vi "Set WordWrap.vi"(8 "error in":errorcluster, 10 "WordWrap":bool, 11 "View in":refnum<class "Cell View.lvclass">) -> (0 "error out":errorcluster, 3 "View out":refnum<class "Cell View.lvclass">)   [LabVIEW 2024, in "SourceGrid.lvlib" / "Cell View.lvclass"]
uses:
  Cell View.lvclass
  Cell View.lvclass/Cell View.ctl
  D:/git/Sourcegrid-LabVIEW/dll/SourceGrid.dll
  dll/SourceGrid.dll
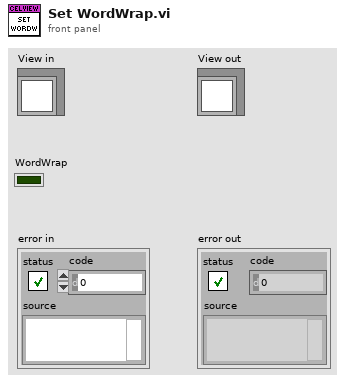
[diagram p1: front panel]
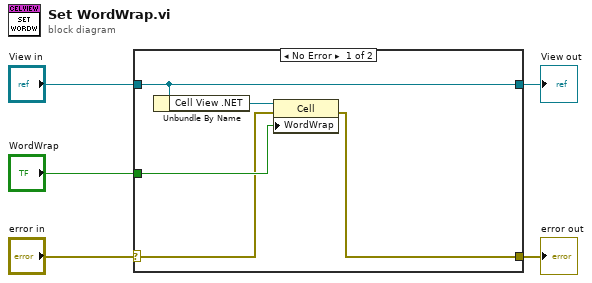
[diagram p0: block diagram]
diagram:
  n1 = case shown="No Error" "error in" {
    selector: "error in" -> [w7 w11]
    tunnel: [w6 w11] -> w4
    tunnel: [w10 w12] -> w2
    tunnel: "View in" -> [w10 w12]
    tunnel: "WordWrap" -> [w8 _]
    frame No Error {
      n2 = Unbundle By Name(w10) -> ("Cell View .NET"=w9:refnum<k24>)
      n3 = property class="Cell"(reference=w9, error in=w7, "WordWrap"=w8) -> (error out=w6:errorcluster)  [unwired: 1 out]
    }
    frame Error {
    }
  }
  "error out" <- w4
  "View out" <- w2
